vi "Generate Async Cmd Event.vi"(7 "AdHoc Cmd (\"\")":string, 8 "error in (no error)":errorcluster, 9 "vData":variant, 10 "AsyncCmd":T1, 11 "Application in":refnum<class "Application.lvclass">) -> (0 "error out":errorcluster, 3 "Application out":refnum<class "Application.lvclass">)   [LabVIEW 2019, in "Application.lvclass"]
doc: "Developed by Kevin Thompson\nkevin@thompsonengineering.net\n\nCopyright 2018\nThompson Engineering, LLC"
uses:
  Application.lvclass
  Common/DataTypes/TD Async CmdMsg EventData--cluster.ctl
  DataTypes/AsynCmd_Application--enum.ctl
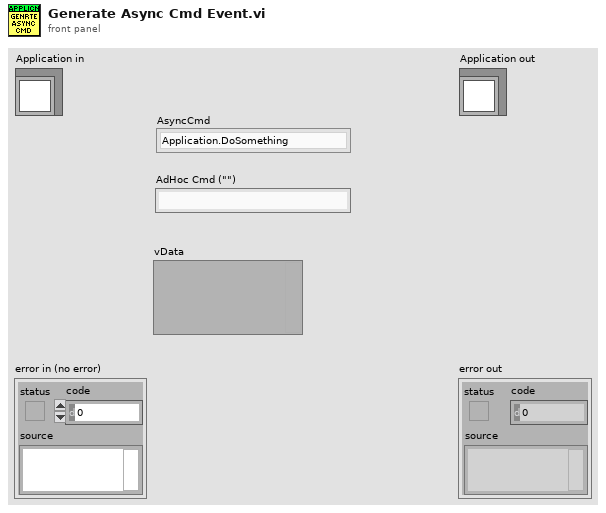
[diagram p1: front panel]
types:
  T1 = typedef "Application.lvclass/AsynCmd_Application--enum.ctl" = enum16{"Application.DoSomething"}
  T2 = typedef "TD Async CmdMsg EventData--cluster.ctl" = cluster{"Time Stamp":timestamp, "CmdMsg":string, "vData":variant}
  T3 = typedef "Application.lvclass/Public Events--cluster.ctl" = cluster{"Application.AsyncCmd Event":refnum<user-event>, "Application.AsyncMsg Event":refnum<user-event>, "stop process":refnum<user-event>}
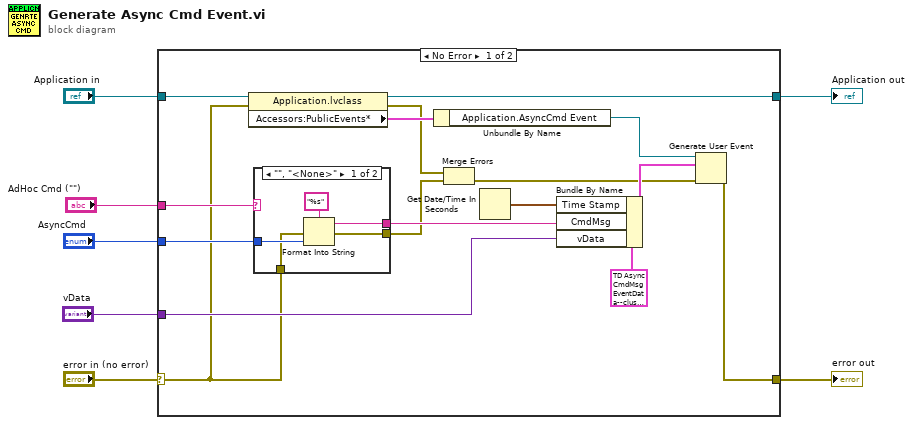
[diagram p0: block diagram]
diagram:
  n1 = case shown="No Error" "error in (no error)" {
    selector: "error in (no error)" -> [w8 w32]
    tunnel: [w23 w32] -> w6
    tunnel: [w13 w31] -> w4
    tunnel: "Application in" -> [w17 w31]
    tunnel: "AsyncCmd" -> [w15 _]
    tunnel: "vData" -> [w18 _]
    tunnel: "AdHoc Cmd (\"\")" -> [w14 _]
    frame No Error {
      n2 = property class="Application.lvclass"(reference=w17, error in=w8) -> (reference out=w13:refnum<class "Application.lvclass">, error out=w10:errorcluster, "Accessors:PublicEvents*"=w12:T3)
      n3 = case shown="\"\", \"<None>\"" w14 {
        selector: w14 -> [_ w29]
        tunnel: w15 -> [w27 _]
        tunnel: [w26 w29] -> w19
        tunnel: w8 -> [w25 w30]
        tunnel: [w24 w30] -> w16
        frame "", "<None>" {
          n4 = Format Into String(format string="%s", error in=w25, w27) -> (resulting string=w26:string, error out=w24:errorcluster)  [unwired: 1 in]
        }
        frame Default {
        }
      }
      n5 = Unbundle By Name(w12) -> ("Application.AsyncCmd Event"=w9:refnum<user-event>)
      n6 = Merge Errors(w10, w16) -> (w11:errorcluster)
      n7 = Get Date/Time In Seconds() -> (seconds since 1Jan1904=w20:timestamp)
      n8 = Bundle By Name(cluster=T2 {"Time Stamp"=timestamp(0 s since 1904-01-01), "CmdMsg"="", "vData"=variant} ("Async EvData"), "Time Stamp"=w20, "CmdMsg"=w19, "vData"=w18) -> (w22:T2)
      n9 = Generate User Event(user event=w9, event data cluster=w22, error in=w11) -> (error out=w23:errorcluster)  [unwired: 1 in, 1 out]
    }
    frame Error {
    }
  }
  "error out" <- w6
  "Application out" <- w4
